vi "update_array_data_and_list_view.vi"(4 "Cmd Pool 2":refnum<vi>, 5 "Cmd Pool 2 List View":refnum<vi>, 6 "Cmd Pool 1":refnum<vi>, 9 "Cmd Array 2":string[](array[string]), 10 "Cmd Array 1":string[](array[string])) -> (0 "Cmd Pool 1 Ref Out":refnum<vi>)   [LabVIEW 2018]
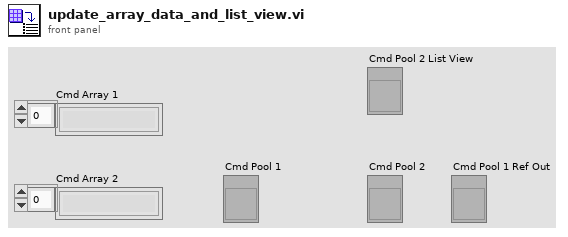
[diagram p1: front panel]
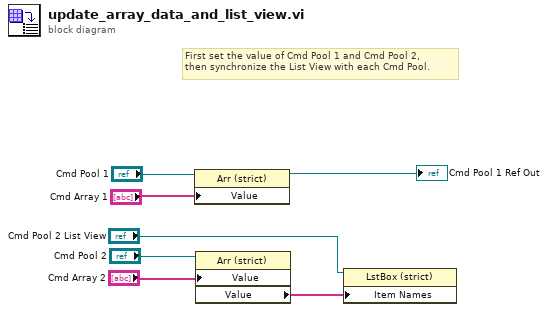
[diagram p0: block diagram]
diagram:
  # "First set the value of Cmd Pool 1 and Cmd Pool 2, \nthen synchronize the List View with each Cmd Pool."
  n1 = property class="Arr (strict)"(reference="Cmd Pool 1", "Value"="Cmd Array 1") -> (reference out=→"Cmd Pool 1 Ref Out":refnum<vi>)  [unwired: 1 in, 1 out]
  n2 = property class="Arr (strict)"(reference="Cmd Pool 2", "Value"="Cmd Array 2") -> ("Value"=w2:string[])  [unwired: 1 in, 2 out]
  n3 = property class="LstBox (strict)"(reference="Cmd Pool 2 List View", "Item Names"=w2) -> ()  [unwired: 1 in, 2 out]
